vi "DGHD5331.vi"() -> ()   [LabVIEW 2014]
uses:
  <vilib>/Instr/_visa.llb/VISA Configure Serial Port (Instr).vi
  <vilib>/Utility/file.llb/Write To Spreadsheet File (string).vi
  <vilib>/Utility/file.llb/Write To Spreadsheet File (DBL).vi
panel:
  in  "Bytes Read":u32
  out "Waveform Chart":cluster{i32, i32, i32, i32}(graph)
  out "concatenated string":string
  out "x*y":dbl
  out "return count":u32
  in  "VISA resource name":refnum<visa-resource-name>
  in  "Loop Timer":u32=500 min=500 max=5000 step=500
  in  "stop":bool
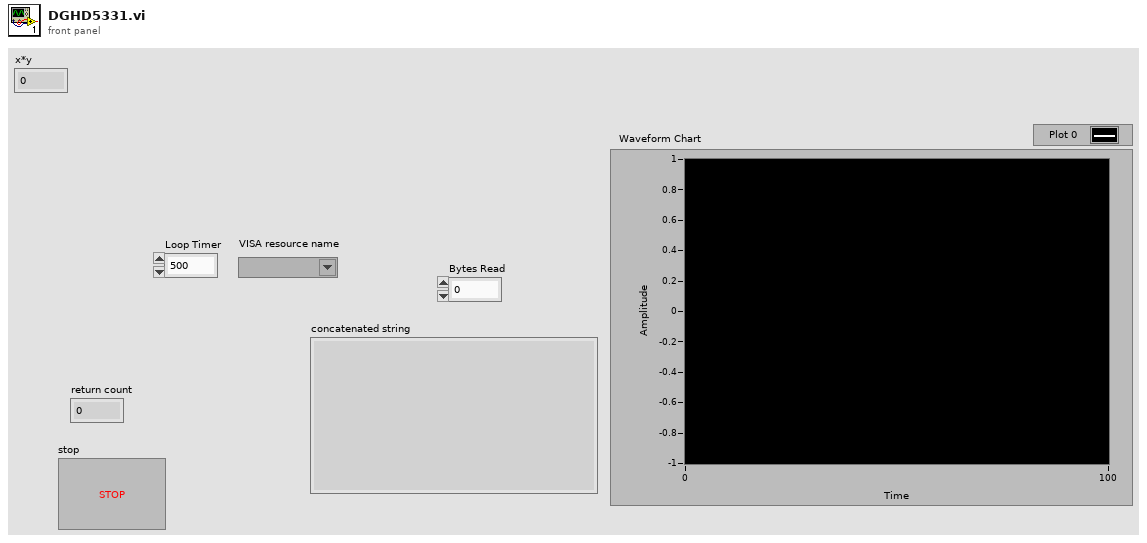
[diagram p1: front panel]
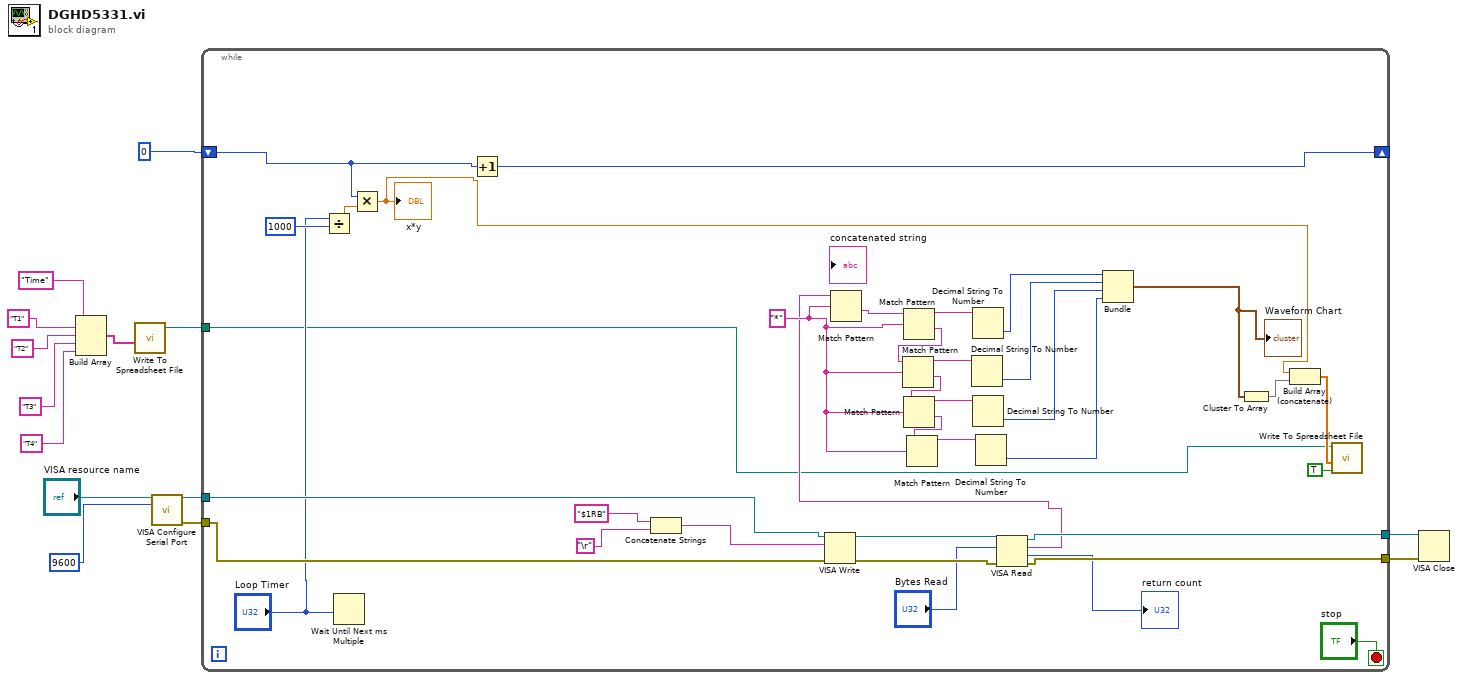
[diagram p0: block diagram]
diagram:
  n1 = Build Array("Time", "T1", "T2", "T3", "T4") -> (w3:string[])
  n2 = call-poly <vilib>:"Write To Spreadsheet File.vi"("1D data"=w3) -> ("new file path (Not A Path if cancelled)"=w1:path)  [unwired: 7 in]
  n3 = call-poly "VISA Configure Serial Port"("VISA resource name"="VISA resource name", "baud rate (9600)"=9600) -> ("VISA resource name out"=w13:refnum<visa-resource-name>, "error out"=w11:errorcluster)  [unwired: 12 in]
  n4 = while {
    tunnel: w13 -> [w50]
    tunnel: w11 -> [w49]
    tunnel: [w46] -> w10
    tunnel: [w45] -> w9
    shift-right: [w18] -> _
    shift-left: 0 -> [w37]
    tunnel: w1 -> [w16]
    stop <- "stop" stop-if-true
    w29 = "*"
    n5 = Divide(x="Loop Timer", y=1000) -> (x/y=w39:dbl)
    n6 = Wait Until Next ms Multiple(millisecond multiple="Loop Timer") -> ()  [unwired: 1 out]
    n7 = Multiply(x=w37, y=w39) -> (x*y=w17:dbl)
    "x*y" <- w17
    n8 = Increment(x=w37) -> (x+1=w18:i32)
    n9 = Concatenate Strings("$1RB", "\r") -> (w41:string)
    n10 = VISA Write(VISA resource name=w50, write buffer=w41, error in (no error)=w49) -> (VISA resource name out=w48:refnum<visa-resource-name>, error out=w47:errorcluster)  [unwired: 1 out]
    n11 = VISA Read(VISA resource name=w48, byte count="Bytes Read", error in (no error)=w47) -> (VISA resource name out=w46:refnum<visa-resource-name>, read buffer=w24:string, return count=→"return count":u32, error out=w45:errorcluster)
    n12 = Match Pattern(string=w24, regular expression=w29) -> (after substring=w36:string)  [unwired: 1 in, 3 out]
    n13 = Match Pattern(string=w36, regular expression=w29) -> (before substring=w35:string, after substring=w33:string)  [unwired: 1 in, 2 out]
    n14 = Match Pattern(string=w33, regular expression=w29) -> (before substring=w34:string, after substring=w28:string)  [unwired: 1 in, 2 out]
    n15 = Match Pattern(string=w28, regular expression=w29) -> (before substring=w31:string, after substring=w27:string)  [unwired: 1 in, 2 out]
    n16 = Match Pattern(string=w27, regular expression=w29) -> (before substring=w30:string)  [unwired: 1 in, 3 out]
    n17 = Decimal String To Number(string=w34) -> (number=w32:i32)  [unwired: 2 in, 1 out]
    n18 = Decimal String To Number(string=w35) -> (number=w23:i32)  [unwired: 2 in, 1 out]
    n19 = Decimal String To Number(string=w31) -> (number=w26:i32)  [unwired: 2 in, 1 out]
    n20 = Decimal String To Number(string=w30) -> (number=w25:i32)  [unwired: 2 in, 1 out]
    n21 = Bundle(w23, w32, w26, w25) -> (w19:cluster{i32, i32, i32, i32})  [unwired: 1 in]
    "Waveform Chart" <- w19
    n22 = Cluster To Array(cluster=w19) -> (array=w21:i32[])
    n23 = Build Array (concatenate)(w17, w21) -> (w20:dbl[])
    n24 = call-poly <vilib>:"Write To Spreadsheet File.vi"("append to file? (new file:F)"=TRUE, "1D data"=w20, "file path (dialog if empty)"=w16) -> ()  [unwired: 5 in, 1 out]
  }
  n25 = VISA Close(VISA resource name=w10, error in (no error)=w9) -> ()  [unwired: 1 out]
